vi "Write configuration.vi"(8 "error in":errorcluster, 10 "configuration":refnum<class "NISE_CEF_serializable configuration.lvclass">, 11 "bin datalogger editor node in":refnum<class "Binary datalogger editor node.lvclass">) -> (0 "error out":errorcluster, 3 "bin datalogger editor node out":refnum<class "Binary datalogger editor node.lvclass">)   [LabVIEW 2013, in "Binary datalogger editor node.lvclass"]
uses:
  Binary datalogger editor node.lvclass
  <vilib>/NI/Configuration Framework/serializable configuration/NISE_CEF_serializable configuration.lvclass
  module/configuration/Binary datalogger configuration.lvclass
  Binary datalogger editor node.lvclass/Binary datalogger editor node.ctl
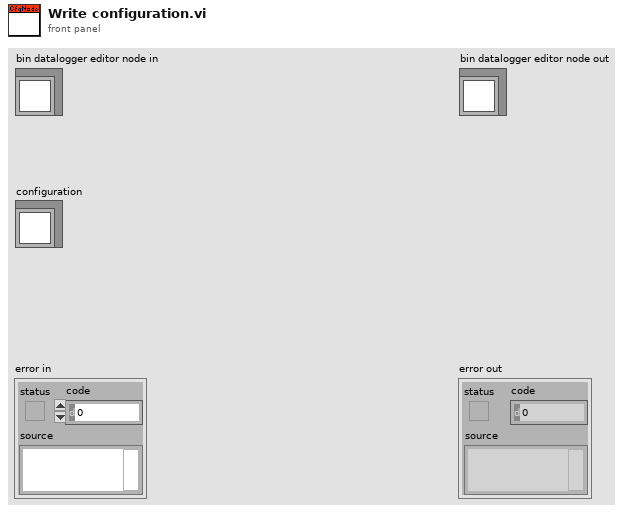
[diagram p1: front panel]
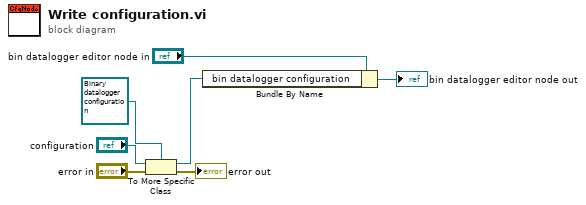
[diagram p0: block diagram]
diagram:
  n1 = To More Specific Class(target class=refnum<class "Binary datalogger configuration.lvclass"> refnum ("bin datalogger configuration"), reference="configuration", error in="error in") -> (specific class reference=w2:refnum<class "Binary datalogger configuration.lvclass">, error out=→"error out":errorcluster)
  n2 = Bundle By Name(cluster="bin datalogger editor node in", "bin datalogger configuration"=w2) -> (→"bin datalogger editor node out":refnum<class "Binary datalogger editor node.lvclass">)
